vi "Lab Panel V4.83.vi"() -> ()   [LabVIEW 2013] (continued)
                            n1243 = local write "data file error"(w2114) -> ()
                          }
                          frame #1 {
                            n1244 = Bundle(cluster=w2115, "STATUS"="T-RISE PASS") -> (w2117:T4)  [unwired: 2 in]
                            n1245 = local write "RESULT LAB03-1"(TRUE) -> ()
                            n1246 = local write "DISP LAB03-1"(w2117) -> ()
                          }
                        }
                      }
                      frame False {
                      }
                    }
                  }
                }
              }
              frame #5 {
                # "LAB03-2"
                n1247 = Equal?(x=w2120, y=2) -> (x = y?=w2123:bool)
                n1248 = local read "DISP LAB03-2"() -> (w2125:T4)
                n1249 = Unbundle(w2125) -> ("STATUS"=w2126:string)  [unwired: 2 out]
                n1250 = Equal?(x=w2126, y="RUN") -> (x = y?=w2122:bool)
                n1251 = And(x=w2122, y=w2123) -> (x .and. y?=w2121:bool)
                n1252 = case shown="True" w2121 {
                  tunnel: w2125 -> [_ w2129]
                  tunnel: w2119 -> [_ w2132]
                  frame False {
                  }
                  frame True {
                    n1253 = local read "SET LAB03-2"() -> (w2131:T5)
                    n1254 = local read "TDMS LAB03-2"() -> (w2128:refnum<k34>)
                    n1255 = Unbundle(w2129) -> ("CYCLE"=w2133:dbl)  [unwired: 2 out]
                    n1256 = Unbundle(w2131) -> ("T-RISE mins"=w2130:dbl)  [unwired: 4 out]
                    n1257 = Greater Or Equal?(x=w2133, y=w2132) -> (x >= y?=w2134:bool)
                    n1258 = case shown="True" w2134 {
                      tunnel: w2130 -> [w2137 _]
                      tunnel: w2129 -> [w2136 _]
                      tunnel: w2128 -> [w2135 _]
                      frame True {
                        n1259 = stacked-sequence {
                          tunnel: w2137 -> [w2140 _]
                          tunnel: w2136 -> [_ w2145]
                          tunnel: w2135 -> [w2138 _]
                          frame #0 {
                            n1260 = Build Array("T-RISE") -> (w2142:string[])
                            n1261 = Build Array(w2140) -> (w2141:dbl[])
                            n1262 = TDMS Write(0:w2138, 5:"TEST PASS", 7:w2142, 9:w2141) -> (15:w2144:errorcluster)  [unwired: 2 in, 3 out]
                            n1263 = local write "data file error"(w2144) -> ()
                          }
                          frame #1 {
                            n1264 = Bundle(cluster=w2145, "STATUS"="T-RISE PASS") -> (w2147:T4)  [unwired: 2 in]
                            n1265 = local write "RESULT LAB03-2"(TRUE) -> ()
                            n1266 = local write "DISP LAB03-2"(w2147) -> ()
                          }
                        }
                      }
                      frame False {
                      }
                    }
                  }
                }
              }
              frame #6 {
                # "LAB04-1"
                n1267 = Equal?(x=w2150, y=2) -> (x = y?=w2153:bool)
                n1268 = local read "DISP LAB04-1"() -> (w2155:T4)
                n1269 = Unbundle(w2155) -> ("STATUS"=w2156:string)  [unwired: 2 out]
                n1270 = Equal?(x=w2156, y="RUN") -> (x = y?=w2152:bool)
                n1271 = And(x=w2152, y=w2153) -> (x .and. y?=w2151:bool)
                n1272 = case shown="True" w2151 {
                  tunnel: w2155 -> [_ w2159]
                  tunnel: w2149 -> [_ w2162]
                  frame False {
                  }
                  frame True {
                    n1273 = local read "SET LAB04-1"() -> (w2161:T5)
                    n1274 = local read "TDMS LAB04-1"() -> (w2158:refnum<k34>)
                    n1275 = Unbundle(w2159) -> ("CYCLE"=w2163:dbl)  [unwired: 2 out]
                    n1276 = Unbundle(w2161) -> ("T-RISE mins"=w2160:dbl)  [unwired: 4 out]
                    n1277 = Greater Or Equal?(x=w2163, y=w2162) -> (x >= y?=w2164:bool)
                    n1278 = case shown="True" w2164 {
                      tunnel: w2160 -> [w2167 _]
                      tunnel: w2159 -> [w2166 _]
                      tunnel: w2158 -> [w2165 _]
                      frame True {
                        n1279 = stacked-sequence {
                          tunnel: w2167 -> [w2170 _]
                          tunnel: w2166 -> [_ w2175]
                          tunnel: w2165 -> [w2168 _]
                          frame #0 {
                            n1280 = Build Array("T-RISE") -> (w2172:string[])
                            n1281 = Build Array(w2170) -> (w2171:dbl[])
                            n1282 = TDMS Write(0:w2168, 5:"TEST PASS", 7:w2172, 9:w2171) -> (15:w2174:errorcluster)  [unwired: 2 in, 3 out]
                            n1283 = local write "data file error"(w2174) -> ()
                          }
                          frame #1 {
                            n1284 = Bundle(cluster=w2175, "STATUS"="T-RISE PASS") -> (w2177:T4)  [unwired: 2 in]
                            n1285 = local write "RESULT LAB04-1"(TRUE) -> ()
                            n1286 = local write "DISP LAB04-1"(w2177) -> ()
                          }
                        }
                      }
                      frame False {
                      }
                    }
                  }
                }
              }
              frame #7 {
                # "LAB04-2"
                n1287 = Equal?(x=w2180, y=2) -> (x = y?=w2183:bool)
                n1288 = local read "DISP LAB04-2"() -> (w2185:T4)
                n1289 = Unbundle(w2185) -> ("STATUS"=w2186:string)  [unwired: 2 out]
                n1290 = Equal?(x=w2186, y="RUN") -> (x = y?=w2182:bool)
                n1291 = And(x=w2182, y=w2183) -> (x .and. y?=w2181:bool)
                n1292 = case shown="True" w2181 {
                  tunnel: w2185 -> [_ w2189]
                  tunnel: w2179 -> [_ w2192]
                  frame False {
                  }
                  frame True {
                    n1293 = local read "SET LAB04-2"() -> (w2191:T5)
                    n1294 = local read "TDMS LAB04-2"() -> (w2188:refnum<k34>)
                    n1295 = Unbundle(w2189) -> ("CYCLE"=w2193:dbl)  [unwired: 2 out]
                    n1296 = Unbundle(w2191) -> ("T-RISE mins"=w2190:dbl)  [unwired: 4 out]
                    n1297 = Greater Or Equal?(x=w2193, y=w2192) -> (x >= y?=w2194:bool)
                    n1298 = case shown="True" w2194 {
                      tunnel: w2190 -> [w2197 _]
                      tunnel: w2189 -> [w2196 _]
                      tunnel: w2188 -> [w2195 _]
                      frame True {
                        n1299 = stacked-sequence {
                          tunnel: w2197 -> [w2200 _]
                          tunnel: w2196 -> [_ w2205]
                          tunnel: w2195 -> [w2198 _]
                          frame #0 {
                            n1300 = Build Array("T-RISE") -> (w2202:string[])
                            n1301 = Build Array(w2200) -> (w2201:dbl[])
                            n1302 = TDMS Write(0:w2198, 5:"TEST PASS", 7:w2202, 9:w2201) -> (15:w2204:errorcluster)  [unwired: 2 in, 3 out]
                            n1303 = local write "data file error"(w2204) -> ()
                          }
                          frame #1 {
                            n1304 = Bundle(cluster=w2205, "STATUS"="T-RISE PASS") -> (w2207:T4)  [unwired: 2 in]
                            n1305 = local write "RESULT LAB04-2"(TRUE) -> ()
                            n1306 = local write "DISP LAB04-2"(w2207) -> ()
                          }
                        }
                      }
                      frame False {
                      }
                    }
                  }
                }
              }
              frame #8 {
                # "LAB05-1"
                n1307 = Equal?(x=w2210, y=2) -> (x = y?=w2213:bool)
                n1308 = local read "DISP LAB05-1"() -> (w2215:T4)
                n1309 = Unbundle(w2215) -> ("STATUS"=w2216:string)  [unwired: 2 out]
                n1310 = Equal?(x=w2216, y="RUN") -> (x = y?=w2212:bool)
                n1311 = And(x=w2212, y=w2213) -> (x .and. y?=w2211:bool)
                n1312 = case shown="True" w2211 {
                  tunnel: w2215 -> [_ w2219]
                  tunnel: w2209 -> [_ w2222]
                  frame False {
                  }
                  frame True {
                    n1313 = local read "SET LAB05-1"() -> (w2221:T5)
                    n1314 = local read "TDMS LAB05-1"() -> (w2218:refnum<k34>)
                    n1315 = Unbundle(w2219) -> ("CYCLE"=w2223:dbl)  [unwired: 2 out]
                    n1316 = Unbundle(w2221) -> ("T-RISE mins"=w2220:dbl)  [unwired: 4 out]
                    n1317 = Greater Or Equal?(x=w2223, y=w2222) -> (x >= y?=w2224:bool)
                    n1318 = case shown="True" w2224 {
                      tunnel: w2220 -> [w2227 _]
                      tunnel: w2219 -> [w2226 _]
                      tunnel: w2218 -> [w2225 _]
                      frame True {
                        n1319 = stacked-sequence {
                          tunnel: w2227 -> [w2230 _]
                          tunnel: w2226 -> [_ w2235]
                          tunnel: w2225 -> [w2228 _]
                          frame #0 {
                            n1320 = Build Array("T-RISE") -> (w2232:string[])
                            n1321 = Build Array(w2230) -> (w2231:dbl[])
                            n1322 = TDMS Write(0:w2228, 5:"TEST PASS", 7:w2232, 9:w2231) -> (15:w2234:errorcluster)  [unwired: 2 in, 3 out]
                            n1323 = local write "data file error"(w2234) -> ()
                          }
                          frame #1 {
                            n1324 = Bundle(cluster=w2235, "STATUS"="T-RISE PASS") -> (w2237:T4)  [unwired: 2 in]
                            n1325 = local write "RESULT LAB05-1"(TRUE) -> ()
                            n1326 = local write "DISP LAB05-1"(w2237) -> ()
                          }
                        }
                      }
                      frame False {
                      }
                    }
                  }
                }
              }
              frame #9 {
                # "LAB05-2"
                n1327 = Equal?(x=w2240, y=2) -> (x = y?=w2243:bool)
                n1328 = local read "DISP LAB05-2"() -> (w2245:T4)
                n1329 = Unbundle(w2245) -> ("STATUS"=w2246:string)  [unwired: 2 out]
                n1330 = Equal?(x=w2246, y="RUN") -> (x = y?=w2242:bool)
                n1331 = And(x=w2242, y=w2243) -> (x .and. y?=w2241:bool)
                n1332 = case shown="True" w2241 {
                  tunnel: w2245 -> [_ w2249]
                  tunnel: w2239 -> [_ w2252]
                  frame False {
                  }
                  frame True {
                    n1333 = local read "SET LAB05-2"() -> (w2251:T5)
                    n1334 = local read "TDMS LAB05-2"() -> (w2248:refnum<k34>)
                    n1335 = Unbundle(w2249) -> ("CYCLE"=w2253:dbl)  [unwired: 2 out]
                    n1336 = Unbundle(w2251) -> ("T-RISE mins"=w2250:dbl)  [unwired: 4 out]
                    n1337 = Greater Or Equal?(x=w2253, y=w2252) -> (x >= y?=w2254:bool)
                    n1338 = case shown="True" w2254 {
                      tunnel: w2250 -> [w2257 _]
                      tunnel: w2249 -> [w2256 _]
                      tunnel: w2248 -> [w2255 _]
                      frame True {
                        n1339 = stacked-sequence {
                          tunnel: w2257 -> [w2260 _]
                          tunnel: w2256 -> [_ w2265]
                          tunnel: w2255 -> [w2258 _]
                          frame #0 {
                            n1340 = Build Array("T-RISE") -> (w2262:string[])
                            n1341 = Build Array(w2260) -> (w2261:dbl[])
                            n1342 = TDMS Write(0:w2258, 5:"TEST PASS", 7:w2262, 9:w2261) -> (15:w2264:errorcluster)  [unwired: 2 in, 3 out]
                            n1343 = local write "data file error"(w2264) -> ()
                          }
                          frame #1 {
                            n1344 = Bundle(cluster=w2265, "STATUS"="T-RISE PASS") -> (w2267:T4)  [unwired: 2 in]
                            n1345 = local write "RESULT LAB05-2"(TRUE) -> ()
                            n1346 = local write "DISP LAB05-2"(w2267) -> ()
                          }
                        }
                      }
                      frame False {
                      }
                    }
                  }
                }
              }
            }
          }
          frame #6 {
            # "end test & close test files"
            n1347 = stacked-sequence {
              tunnel: w2278 -> [_ _ _ _ _ _ _ _ _ _]
              tunnel: w2279 -> [_ _ _ _ _ _ _ _ _ _]
              tunnel: w2277 -> [_ _ _ _ _ _ _ _ _ _]
              tunnel: w2276 -> [_ _ _ _ _ _ _ _ _ _]
              tunnel: w2275 -> [_ _ _ _ _ _ _ _ _ _]
              tunnel: w2274 -> [_ _ _ _ _ _ _ _ _ _]
              tunnel: w2273 -> [_ _ _ _ _ _ _ _ _ _]
              tunnel: w2272 -> [_ _ _ _ _ _ _ _ _ _]
              tunnel: w2271 -> [_ _ _ _ _ _ _ _ _ _]
              tunnel: w2270 -> [_ _ _ _ _ _ _ _ _ _]
              frame #0 {
                # "LAB01-1"
                n1348 = local read "DISP LAB01-1"() -> (w2283:T4)
                n1349 = local read "run lab01-1"() -> (w2280:bool)
                n1350 = local read "TDMS LAB01-1"() -> (w2281:refnum<k34>)
                n1351 = Unbundle(w2283) -> ("CYCLE"=w2284:dbl, "STATUS"=w2282:string)  [unwired: 1 out]
                n1352 = case shown="True" w2280 {
                  tunnel: w2284 -> [_ w2285]
                  tunnel: w2283 -> [_ w2288]
                  tunnel: w2282 -> [_ w2287]
                  tunnel: w2281 -> [_ w2286]
                  frame False {
                  }
                  frame True {
                    n1353 = Not Equal?(x=w2287, y="RUN") -> (x != y?=w2289:bool)
                    n1354 = Greater?(x=w2285, y=2.0) -> (0:w2291:bool)
                    n1355 = And(x=w2291, y=w2289) -> (x .and. y?=w2290:bool)
                    n1356 = case shown="True" w2290 {
                      tunnel: w2288 -> [_ w2296]
                      tunnel: w2286 -> [_ w2295]
                      tunnel: w2285 -> [_ w2294]
                      frame False {
                      }
                      frame True {
                        n1357 = stacked-sequence {
                          tunnel: w2296 -> [w2300 _ _]
                          tunnel: w2295 -> [_ w2302 _]
                          tunnel: w2294 -> [_ _ _]
                          frame #0 {
                            w2297 = FALSE
                            n1358 = local write "mail control"("END") -> ()
                            n1359 = Bundle(cluster=w2300) -> (w2299:T4)  [unwired: 3 in]
                            n1360 = local write "DISP LAB01-1"(w2299) -> ()
                            n1361 = local write "O/I  LAB01-1"(w2297) -> ()
                            n1362 = local write "run lab01-1"(w2297) -> ()
                            n1363 = local write "RUN LAB01-1"(w2297) -> ()
                          }
                          frame #1 {
                            n1364 = TDMS Close(11:w2302) -> (0:w2301:errorcluster)  [unwired: 1 in, 1 out]
                            n1365 = local write "data file error"(w2301) -> ()
                          }
                          frame #2 {
                            n1366 = stacked-sequence {
                              tunnel: "LAB01-1" -> [w2305 w2307]
                              frame #0 {
                                n1367 = call "sub vi - defrag tdms v1.vi"("panel id"=w2305) -> ("error out"=w2304:errorcluster)  [unwired: 10 in]
                                n1368 = local write "data file error"(w2304) -> ()
                              }
                              frame #1 {
                                n1369 = call "Save data file to network drive v2.vi"("panel id"=w2307) -> ("network file save error"=w2306:errorcluster)  [unwired: 9 in, 1 out]
                                n1370 = local write "data file error"(w2306) -> ()
                              }
                            }
                          }
                        }
                      }
                    }
                  }
                }
              }
              frame #1 {
                # "LAB01-2"
                n1371 = local read "run lab01-2"() -> (w2308:bool)
                n1372 = case shown="True" w2308 {
                  frame False {
                  }
                  frame True {
                    n1373 = local read "DISP LAB01-2"() -> (w2315:T4)
                    n1374 = local read "TDMS LAB01-2"() -> (w2314:refnum<k34>)
                    n1375 = Unbundle(w2315) -> ("CYCLE"=w2309:dbl, "STATUS"=w2316:string)  [unwired: 1 out]
                    n1376 = Not Equal?(x=w2316, y="RUN") -> (x != y?=w2311:bool)
                    n1377 = Greater?(x=w2309, y=2.0) -> (0:w2312:bool)
                    n1378 = And(x=w2312, y=w2311) -> (x .and. y?=w2310:bool)
                    n1379 = case shown="True" w2310 {
                      tunnel: w2315 -> [_ w2320]
                      tunnel: w2314 -> [_ w2319]
                      tunnel: w2309 -> [_ w2318]
                      frame False {
                      }
                      frame True {
                        n1380 = stacked-sequence {
                          tunnel: w2320 -> [w2323 _ _]
                          tunnel: w2319 -> [_ w2325 _]
                          tunnel: w2318 -> [_ _ _]
                          frame #0 {
                            w2321 = FALSE
                            n1381 = local write "mail control"("END") -> ()
                            n1382 = Bundle(cluster=w2323) -> (w2324:T4)  [unwired: 3 in]
                            n1383 = local write "RUN LAB01-2"(w2321) -> ()
                            n1384 = local write "run lab01-2"(w2321) -> ()
                            n1385 = local write "O/I  LAB01-2"(w2321) -> ()
                            n1386 = local write "DISP LAB01-2"(w2324) -> ()
                          }
                          frame #1 {
                            n1387 = TDMS Close(11:w2325) -> (0:w2326:errorcluster)  [unwired: 1 in, 1 out]
                            n1388 = local write "data file error"(w2326) -> ()
                          }
                          frame #2 {
                            n1389 = stacked-sequence {
                              tunnel: "LAB01-2" -> [w2329 w2331]
                              frame #0 {
                                n1390 = call "sub vi - defrag tdms v1.vi"("panel id"=w2329) -> ("error out"=w2328:errorcluster)  [unwired: 10 in]
                                n1391 = local write "data file error"(w2328) -> ()
                              }
                              frame #1 {
                                n1392 = call "Save data file to network drive v2.vi"("panel id"=w2331) -> ("network file save error"=w2330:errorcluster)  [unwired: 9 in, 1 out]
                                n1393 = local write "data file error"(w2330) -> ()
                              }
                            }
                          }
                        }
                      }
                    }
                  }
                }
              }
              frame #2 {
                # "LAB02-1"
                n1394 = local read "run lab02-1"() -> (w2332:bool)
                n1395 = case shown="True" w2332 {
                  frame False {
                  }
                  frame True {
                    n1396 = local read "DISP LAB02-1"() -> (w2339:T4)
                    n1397 = Unbundle(w2339) -> ("CYCLE"=w2335:dbl, "STATUS"=w2340:string)  [unwired: 1 out]
                    n1398 = local read "TDMS LAB02-1"() -> (w2338:refnum<k34>)
                    n1399 = Not Equal?(x=w2340, y="RUN") -> (x != y?=w2334:bool)
                    n1400 = Greater?(x=w2335, y=2.0) -> (0:w2336:bool)
                    n1401 = And(x=w2336, y=w2334) -> (x .and. y?=w2333:bool)
                    n1402 = case shown="True" w2333 {
                      tunnel: w2339 -> [_ w2343]
                      tunnel: w2338 -> [_ w2342]
                      frame False {
                      }
                      frame True {
                        n1403 = stacked-sequence {
                          tunnel: w2343 -> [w2346 _ _]
                          tunnel: w2342 -> [_ w2348 _]
                          frame #0 {
                            w2344 = FALSE
                            n1404 = local write "mail control"("END") -> ()
                            n1405 = Bundle(cluster=w2346) -> (w2347:T4)  [unwired: 3 in]
                            n1406 = local write "O/I  LAB02-1"(w2344) -> ()
                            n1407 = local write "RUN LAB02-1"(w2344) -> ()
                            n1408 = local write "run lab02-1"(w2344) -> ()
                            n1409 = local write "DISP LAB02-1"(w2347) -> ()
                          }
                          frame #1 {
                            n1410 = TDMS Close(11:w2348) -> (0:w2349:errorcluster)  [unwired: 1 in, 1 out]
                            n1411 = local write "data file error"(w2349) -> ()
                          }
                          frame #2 {
                            n1412 = stacked-sequence {
                              tunnel: "LAB02-1" -> [w2352 w2354]
                              frame #0 {
                                n1413 = call "sub vi - defrag tdms v1.vi"("panel id"=w2352) -> ("error out"=w2351:errorcluster)  [unwired: 10 in]
                                n1414 = local write "data file error"(w2351) -> ()
                              }
                              frame #1 {
                                n1415 = call "Save data file to network drive v2.vi"("panel id"=w2354) -> ("network file save error"=w2353:errorcluster)  [unwired: 9 in, 1 out]
                                n1416 = local write "data file error"(w2353) -> ()
                              }
                            }
                          }
                        }
                      }
                    }
                  }
                }
              }
              frame #3 {
                # "LAB02-2"
                n1417 = local read "run lab02-2"() -> (w2355:bool)
                n1418 = case shown="True" w2355 {
                  frame False {
                  }
                  frame True {
                    n1419 = local read "DISP LAB02-2"() -> (w2362:T4)
                    n1420 = local read "TDMS LAB02-2"() -> (w2361:refnum<k34>)
                    n1421 = Unbundle(w2362) -> ("CYCLE"=w2358:dbl, "STATUS"=w2363:string)  [unwired: 1 out]
                    n1422 = Not Equal?(x=w2363, y="RUN") -> (x != y?=w2357:bool)
                    n1423 = Greater?(x=w2358, y=2.0) -> (0:w2359:bool)
                    n1424 = And(x=w2359, y=w2357) -> (x .and. y?=w2356:bool)
                    n1425 = case shown="True" w2356 {
                      tunnel: w2362 -> [_ w2366]
                      tunnel: w2361 -> [_ w2365]
                      frame False {
                      }
                      frame True {
                        n1426 = stacked-sequence {
                          tunnel: w2366 -> [w2369 _ _]
                          tunnel: w2365 -> [_ w2371 _]
                          frame #0 {
                            w2367 = FALSE
                            n1427 = local write "mail control"("END") -> ()
                            n1428 = Bundle(cluster=w2369) -> (w2370:T4)  [unwired: 3 in]
                            n1429 = local write "O/I  LAB02-2"(w2367) -> ()
                            n1430 = local write "run lab02-2"(w2367) -> ()
                            n1431 = local write "RUN LAB02-2"(w2367) -> ()
                            n1432 = local write "DISP LAB02-2"(w2370) -> ()
                          }
                          frame #1 {
                            n1433 = TDMS Close(11:w2371) -> (0:w2372:errorcluster)  [unwired: 1 in, 1 out]
                            n1434 = local write "data file error"(w2372) -> ()
                          }
                          frame #2 {
                            n1435 = stacked-sequence {
                              tunnel: "LAB02-2" -> [w2375 w2377]
                              frame #0 {
                                n1436 = call "sub vi - defrag tdms v1.vi"("panel id"=w2375) -> ("error out"=w2374:errorcluster)  [unwired: 10 in]
                                n1437 = local write "data file error"(w2374) -> ()
                              }
                              frame #1 {
                                n1438 = call "Save data file to network drive v2.vi"("panel id"=w2377) -> ("network file save error"=w2376:errorcluster)  [unwired: 9 in, 1 out]
                                n1439 = local write "data file error"(w2376) -> ()
                              }
                            }
                          }
                        }
                      }
                    }
                  }
                }
              }
              frame #4 {
                # "LAB03-1"
                n1440 = local read "run lab03-1"() -> (w2378:bool)
                n1441 = case shown="True" w2378 {
                  frame False {
                  }
                  frame True {
                    n1442 = local read "DISP LAB03-1"() -> (w2385:T4)
                    n1443 = local read "TDMS LAB03-1"() -> (w2384:refnum<k34>)
                    n1444 = Unbundle(w2385) -> ("CYCLE"=w2381:dbl, "STATUS"=w2386:string)  [unwired: 1 out]
                    n1445 = Not Equal?(x=w2386, y="RUN") -> (x != y?=w2380:bool)
                    n1446 = Greater?(x=w2381, y=2.0) -> (0:w2382:bool)
                    n1447 = And(x=w2382, y=w2380) -> (x .and. y?=w2379:bool)
                    n1448 = case shown="True" w2379 {
                      tunnel: w2385 -> [_ w2389]
                      tunnel: w2384 -> [_ w2388]
                      frame False {
                      }
                      frame True {
                        n1449 = stacked-sequence {
                          tunnel: w2389 -> [w2392 _ _]
                          tunnel: w2388 -> [_ w2394 _]
                          frame #0 {
                            w2390 = FALSE
                            n1450 = local write "mail control"("END") -> ()
                            n1451 = Bundle(cluster=w2392) -> (w2393:T4)  [unwired: 3 in]
                            n1452 = local write "O/I  LAB03-1"(w2390) -> ()
                            n1453 = local write "run lab03-1"(w2390) -> ()
                            n1454 = local write "RUN LAB03-1"(w2390) -> ()
                            n1455 = local write "DISP LAB03-1"(w2393) -> ()
                          }
                          frame #1 {
                            n1456 = TDMS Close(11:w2394) -> (0:w2395:errorcluster)  [unwired: 1 in, 1 out]
                            n1457 = local write "data file error"(w2395) -> ()
                          }
                          frame #2 {
                            n1458 = stacked-sequence {
                              tunnel: "LAB03-1" -> [w2398 w2400]
                              frame #0 {
                                n1459 = call "sub vi - defrag tdms v1.vi"("panel id"=w2398) -> ("error out"=w2397:errorcluster)  [unwired: 10 in]
                                n1460 = local write "data file error"(w2397) -> ()
                              }
                              frame #1 {
                                n1461 = call "Save data file to network drive v2.vi"("panel id"=w2400) -> ("network file save error"=w2399:errorcluster)  [unwired: 9 in, 1 out]
                                n1462 = local write "data file error"(w2399) -> ()
                              }
                            }
                          }
                        }
                      }
                    }
                  }
                }
              }
              frame #5 {
                # "LAB03-2"
                n1463 = local read "run lab03-2"() -> (w2401:bool)
                n1464 = case shown="True" w2401 {
                  frame False {
                  }
                  frame True {
                    n1465 = local read "DISP LAB03-2"() -> (w2408:T4)
                    n1466 = Unbundle(w2408) -> ("CYCLE"=w2404:dbl, "STATUS"=w2409:string)  [unwired: 1 out]
                    n1467 = local read "TDMS LAB03-2"() -> (w2407:refnum<k34>)
                    n1468 = Not Equal?(x=w2409, y="RUN") -> (x != y?=w2403:bool)
                    n1469 = Greater?(x=w2404, y=2.0) -> (0:w2405:bool)
                    n1470 = And(x=w2405, y=w2403) -> (x .and. y?=w2402:bool)
                    n1471 = case shown="True" w2402 {
                      tunnel: w2408 -> [_ w2412]
                      tunnel: w2407 -> [_ w2411]
                      frame False {
                      }
                      frame True {
                        n1472 = stacked-sequence {
                          tunnel: w2412 -> [w2415 _ _]
                          tunnel: w2411 -> [_ w2417 _]
                          frame #0 {
                            w2413 = FALSE
                            n1473 = local write "mail control"("END") -> ()
                            n1474 = Bundle(cluster=w2415) -> (w2416:T4)  [unwired: 3 in]
                            n1475 = local write "RUN LAB03-2"(w2413) -> ()
                            n1476 = local write "O/I  LAB03-2"(w2413) -> ()
                            n1477 = local write "DISP LAB03-2"(w2416) -> ()
                            n1478 = local write "run lab03-2"(w2413) -> ()
                          }
                          frame #1 {
                            n1479 = TDMS Close(11:w2417) -> (0:w2418:errorcluster)  [unwired: 1 in, 1 out]
                            n1480 = local write "data file error"(w2418) -> ()
                          }
                          frame #2 {
                            n1481 = stacked-sequence {
                              tunnel: "LAB03-2" -> [w2421 w2423]
                              frame #0 {
                                n1482 = call "sub vi - defrag tdms v1.vi"("panel id"=w2421) -> ("error out"=w2420:errorcluster)  [unwired: 10 in]
                                n1483 = local write "data file error"(w2420) -> ()
                              }
                              frame #1 {
                                n1484 = call "Save data file to network drive v2.vi"("panel id"=w2423) -> ("network file save error"=w2422:errorcluster)  [unwired: 9 in, 1 out]
                                n1485 = local write "data file error"(w2422) -> ()
                              }
                            }
                          }
                        }
                      }
                    }
                  }
                }
              }
              frame #6 {
                # "LAB04-1"
                n1486 = local read "run lab04-1"() -> (w2424:bool)
                n1487 = case shown="True" w2424 {
                  frame False {
                  }
                  frame True {
                    n1488 = local read "DISP LAB04-1"() -> (w2431:T4)
                    n1489 = Unbundle(w2431) -> ("CYCLE"=w2427:dbl, "STATUS"=w2432:string)  [unwired: 1 out]
                    n1490 = local read "TDMS LAB04-1"() -> (w2430:refnum<k34>)
                    n1491 = Not Equal?(x=w2432, y="RUN") -> (x != y?=w2426:bool)
                    n1492 = Greater?(x=w2427, y=2.0) -> (0:w2428:bool)
                    n1493 = And(x=w2428, y=w2426) -> (x .and. y?=w2425:bool)
                    n1494 = case shown="True" w2425 {
                      tunnel: w2431 -> [_ w2435]
                      tunnel: w2430 -> [_ w2434]
                      frame False {
                      }
                      frame True {
                        n1495 = stacked-sequence {
                          tunnel: w2435 -> [w2438 _ _]
                          tunnel: w2434 -> [_ w2440 _]
                          frame #0 {
                            w2436 = FALSE
                            n1496 = local write "mail control"("END") -> ()
                            n1497 = Bundle(cluster=w2438) -> (w2439:T4)  [unwired: 3 in]
                            n1498 = local write "RUN LAB04-1"(w2436) -> ()
                            n1499 = local write "O/I  LAB04-1"(w2436) -> ()
                            n1500 = local write "run lab04-1"(w2436) -> ()
                            n1501 = local write "DISP LAB04-1"(w2439) -> ()
                          }
                          frame #1 {
                            n1502 = TDMS Close(11:w2440) -> (0:w2441:errorcluster)  [unwired: 1 in, 1 out]
                            n1503 = local write "data file error"(w2441) -> ()
                          }
                          frame #2 {
                            n1504 = stacked-sequence {
                              tunnel: "LAB04-1" -> [w2444 w2446]
                              frame #0 {
                                n1505 = call "sub vi - defrag tdms v1.vi"("panel id"=w2444) -> ("error out"=w2443:errorcluster)  [unwired: 10 in]
                                n1506 = local write "data file error"(w2443) -> ()
                              }
                              frame #1 {
                                n1507 = call "Save data file to network drive v2.vi"("panel id"=w2446) -> ("network file save error"=w2445:errorcluster)  [unwired: 9 in, 1 out]
                                n1508 = local write "data file error"(w2445) -> ()
                              }
                            }
                          }
                        }
                      }
                    }
                  }
                }
              }
              frame #7 {
                # "LAB04-2"
                n1509 = local read "run lab04-2"() -> (w2447:bool)
                n1510 = case shown="True" w2447 {
                  frame False {
                  }
                  frame True {
                    n1511 = local read "DISP LAB04-2"() -> (w2454:T4)
                    n1512 = Unbundle(w2454) -> ("CYCLE"=w2450:dbl, "STATUS"=w2455:string)  [unwired: 1 out]
                    n1513 = Not Equal?(x=w2455, y="RUN") -> (x != y?=w2449:bool)
                    n1514 = local read "TDMS LAB04-2"() -> (w2453:refnum<k34>)
                    n1515 = Greater?(x=w2450, y=2.0) -> (0:w2451:bool)
                    n1516 = And(x=w2451, y=w2449) -> (x .and. y?=w2448:bool)
                    n1517 = case shown="True" w2448 {
                      tunnel: w2454 -> [_ w2458]
                      tunnel: w2453 -> [_ w2457]
                      frame False {
                      }
                      frame True {
                        n1518 = stacked-sequence {
                          tunnel: w2458 -> [w2461 _ _]
                          tunnel: w2457 -> [_ w2463 _]
                          frame #0 {
                            w2459 = FALSE
                            n1519 = local write "mail control"("END") -> ()
                            n1520 = Bundle(cluster=w2461) -> (w2462:T4)  [unwired: 3 in]
                            n1521 = local write "O/I  LAB04-2"(w2459) -> ()
                            n1522 = local write "RUN LAB04-2"(w2459) -> ()
                            n1523 = local write "run lab04-2"(w2459) -> ()
                            n1524 = local write "DISP LAB04-2"(w2462) -> ()
                          }
                          frame #1 {
                            n1525 = TDMS Close(11:w2463) -> (0:w2464:errorcluster)  [unwired: 1 in, 1 out]
                            n1526 = local write "data file error"(w2464) -> ()
                          }
                          frame #2 {
                            n1527 = stacked-sequence {
                              tunnel: "LAB04-2" -> [w2467 w2469]
                              frame #0 {
                                n1528 = call "sub vi - defrag tdms v1.vi"("panel id"=w2467) -> ("error out"=w2466:errorcluster)  [unwired: 10 in]
                                n1529 = local write "data file error"(w2466) -> ()
                              }
                              frame #1 {
                                n1530 = call "Save data file to network drive v2.vi"("panel id"=w2469) -> ("network file save error"=w2468:errorcluster)  [unwired: 9 in, 1 out]
                                n1531 = local write "data file error"(w2468) -> ()
                              }
                            }
                          }
                        }
                      }
                    }
                  }
                }
              }
              frame #8 {
                # "LAB05-1"
                n1532 = local read "run lab05-1"() -> (w2470:bool)
                n1533 = case shown="True" w2470 {
                  frame False {
                  }
                  frame True {
                    n1534 = local read "DISP LAB05-1"() -> (w2477:T4)
                    n1535 = Unbundle(w2477) -> ("CYCLE"=w2473:dbl, "STATUS"=w2478:string)  [unwired: 1 out]
                    n1536 = Not Equal?(x=w2478, y="RUN") -> (x != y?=w2472:bool)
                    n1537 = local read "TDMS LAB05-1"() -> (w2476:refnum<k34>)
                    n1538 = Greater?(x=w2473, y=2.0) -> (0:w2474:bool)
                    n1539 = And(x=w2474, y=w2472) -> (x .and. y?=w2471:bool)
                    n1540 = case shown="True" w2471 {
                      tunnel: w2477 -> [_ w2481]
                      tunnel: w2476 -> [_ w2480]
                      frame False {
                      }
                      frame True {
                        n1541 = stacked-sequence {
                          tunnel: w2481 -> [w2484 _ _]
                          tunnel: w2480 -> [_ w2486 _]
                          frame #0 {
                            w2482 = FALSE
                            n1542 = local write "mail control"("END") -> ()
                            n1543 = Bundle(cluster=w2484) -> (w2485:T4)  [unwired: 3 in]
                            n1544 = local write "O/I  LAB05-1"(w2482) -> ()
                            n1545 = local write "RUN LAB05-1"(w2482) -> ()
                            n1546 = local write "run lab05-1"(w2482) -> ()
                            n1547 = local write "DISP LAB05-1"(w2485) -> ()
                          }
                          frame #1 {
                            n1548 = TDMS Close(11:w2486) -> (0:w2487:errorcluster)  [unwired: 1 in, 1 out]
                            n1549 = local write "data file error"(w2487) -> ()
                          }
                          frame #2 {
                            n1550 = stacked-sequence {
                              tunnel: "LAB05-1" -> [w2490 w2492]
                              frame #0 {
                                n1551 = call "sub vi - defrag tdms v1.vi"("panel id"=w2490) -> ("error out"=w2489:errorcluster)  [unwired: 10 in]
                                n1552 = local write "data file error"(w2489) -> ()
                              }
                              frame #1 {
                                n1553 = call "Save data file to network drive v2.vi"("panel id"=w2492) -> ("network file save error"=w2491:errorcluster)  [unwired: 9 in, 1 out]
                                n1554 = local write "data file error"(w2491) -> ()
                              }
                            }
                          }
                        }
                      }
                    }
                  }
                }
              }
              frame #9 {
                # "LAB05-2"
                n1555 = local read "run lab05-2"() -> (w2493:bool)
                n1556 = case shown="True" w2493 {
                  frame False {
                  }
                  frame True {
                    n1557 = local read "DISP LAB05-2"() -> (w2500:T4)
                    n1558 = Unbundle(w2500) -> ("CYCLE"=w2496:dbl, "STATUS"=w2501:string)  [unwired: 1 out]
                    n1559 = Not Equal?(x=w2501, y="RUN") -> (x != y?=w2495:bool)
                    n1560 = local read "TDMS LAB05-2"() -> (w2499:refnum<k34>)
                    n1561 = Greater?(x=w2496, y=2.0) -> (0:w2497:bool)
                    n1562 = And(x=w2497, y=w2495) -> (x .and. y?=w2494:bool)
                    n1563 = case shown="True" w2494 {
                      tunnel: w2500 -> [_ w2504]
                      tunnel: w2499 -> [_ w2503]
                      frame False {
                      }
                      frame True {
                        n1564 = stacked-sequence {
                          tunnel: w2504 -> [w2507 _ _]
                          tunnel: w2503 -> [_ w2509 _]
                          frame #0 {
                            w2505 = FALSE
                            n1565 = local write "mail control"("END") -> ()
                            n1566 = Bundle(cluster=w2507) -> (w2508:T4)  [unwired: 3 in]
                            n1567 = local write "RUN LAB05-2"(w2505) -> ()
                            n1568 = local write "O/I  LAB05-2"(w2505) -> ()
                            n1569 = local write "run lab05-2"(w2505) -> ()
                            n1570 = local write "DISP LAB05-2"(w2508) -> ()
                          }
                          frame #1 {
                            n1571 = TDMS Close(11:w2509) -> (0:w2510:errorcluster)  [unwired: 1 in, 1 out]
                            n1572 = local write "data file error"(w2510) -> ()
                          }
                          frame #2 {
                            n1573 = stacked-sequence {
                              tunnel: "LAB05-2" -> [w2513 w2515]
                              frame #0 {
                                n1574 = call "sub vi - defrag tdms v1.vi"("panel id"=w2513) -> ("error out"=w2512:errorcluster)  [unwired: 10 in]
                                n1575 = local write "data file error"(w2512) -> ()
                              }
                              frame #1 {
                                n1576 = call "Save data file to network drive v2.vi"("panel id"=w2515) -> ("network file save error"=w2514:errorcluster)  [unwired: 9 in, 1 out]
                                n1577 = local write "data file error"(w2514) -> ()
                              }
                            }
                          }
                        }
                      }
                    }
                  }
                }
              }
            }
            n1578 = local read "Network Directory"() -> (w2269:path)
            n1579 = global write "Global 1.vi" "Network Drive"(w2269) -> ()
          }
          frame #7 {
            # "disable functions"
            n1580 = stacked-sequence {
              tunnel: w2525 -> [w2539 _ w2596]
              tunnel: w2524 -> [w2534 _ w2595]
              tunnel: w2523 -> [w2533 _ w2594]
              tunnel: w2522 -> [w2531 _ w2593]
              tunnel: w2521 -> [w2532 _ w2592]
              tunnel: w2520 -> [_ w2556 w2591]
              tunnel: w2519 -> [_ w2557 w2590]
              tunnel: w2518 -> [_ w2558 w2589]
              tunnel: w2517 -> [_ w2559 w2588]
              tunnel: w2516 -> [_ w2560 w2587]
              frame #0 {
                n1581 = Select(t=2, s=w2531, f=0) -> (s? t:f=w2527:i32)
                n1582 = Select(t=2, s=w2533, f=0) -> (s? t:f=w2528:i32)
                n1583 = Select(t=2, s=w2532, f=0) -> (s? t:f=w2526:i32)
                n1584 = Select(t=2, s=w2539, f=0) -> (s? t:f=w2530:i32)
                n1585 = Select(t=2, s=w2534, f=0) -> (s? t:f=w2529:i32)
                n1586 = property on="SELECT LAB02-2" class="RadioBtnsControl (strict)"("DisabledEnum"=w2527) -> ()  [unwired: 2 in, 2 out]
                n1587 = property on="SELECT LAB02-1" class="RadioBtnsControl (strict)"("DisabledEnum"=w2528) -> ()  [unwired: 2 in, 2 out]
                n1588 = property on="SELECT LAB03-1" class="RadioBtnsControl (strict)"("DisabledEnum"=w2526) -> ()  [unwired: 2 in, 2 out]
                n1589 = property on="SELECT LAB01-1" class="RadioBtnsControl (strict)"("DisabledEnum"=w2530) -> ()  [unwired: 2 in, 2 out]
                n1590 = property on="SELECT LAB01-2" class="RadioBtnsControl (strict)"("DisabledEnum"=w2529) -> ()  [unwired: 2 in, 2 out]
                n1591 = Not(x=w2539) -> (.not. x?=w2540:bool)
                n1592 = property on="RESULT LAB01-1" class="Bool (strict)"("Visible"=w2540) -> ()  [unwired: 2 in, 2 out]
                n1593 = Not(x=w2534) -> (.not. x?=w2538:bool)
                n1594 = Not(x=w2533) -> (.not. x?=w2537:bool)
                n1595 = Not(x=w2531) -> (.not. x?=w2536:bool)
                n1596 = property on="RESULT LAB01-2" class="Bool (strict)"("Visible"=w2538) -> ()  [unwired: 2 in, 2 out]
                n1597 = Not(x=w2532) -> (.not. x?=w2535:bool)
                n1598 = property on="RESULT LAB02-1" class="Bool (strict)"("Visible"=w2537) -> ()  [unwired: 2 in, 2 out]
                n1599 = property on="RESULT LAB02-2" class="Bool (strict)"("Visible"=w2536) -> ()  [unwired: 2 in, 2 out]
                n1600 = property on="RESULT LAB03-1" class="Bool (strict)"("Visible"=w2535) -> ()  [unwired: 2 in, 2 out]
                n1601 = property on="SET LAB01-1" class="Clust (strict)"("DisabledEnum"=w2530) -> ()  [unwired: 2 in, 2 out]
                n1602 = property on="SET LAB01-2" class="Clust (strict)"("DisabledEnum"=w2529) -> ()  [unwired: 2 in, 2 out]
                n1603 = property on="SET LAB02-1" class="Clust (strict)"("DisabledEnum"=w2528) -> ()  [unwired: 2 in, 2 out]
                n1604 = property on="SET LAB02-2" class="Clust (strict)"("DisabledEnum"=w2527) -> ()  [unwired: 2 in, 2 out]
                n1605 = property on="SET LAB03-1" class="Clust (strict)"("DisabledEnum"=w2526) -> ()  [unwired: 2 in, 2 out]
                n1606 = property on="O/I  LAB01-1" class="Bool (strict)"("DisabledEnum"=w2530) -> ()  [unwired: 2 in, 2 out]
                n1607 = property on="O/I  LAB01-2" class="Bool (strict)"("DisabledEnum"=w2529) -> ()  [unwired: 2 in, 2 out]
                n1608 = property on="O/I  LAB02-1" class="Bool (strict)"("DisabledEnum"=w2528) -> ()  [unwired: 2 in, 2 out]
                n1609 = property on="O/I  LAB02-2" class="Bool (strict)"("DisabledEnum"=w2527) -> ()  [unwired: 2 in, 2 out]
                n1610 = property on="O/I  LAB03-1" class="Bool (strict)"("DisabledEnum"=w2526) -> ()  [unwired: 2 in, 2 out]
              }
              frame #1 {
                n1611 = Select(t=2, s=w2560, f=0) -> (s? t:f=w2551:i32)
                n1612 = Select(t=2, s=w2559, f=0) -> (s? t:f=w2552:i32)
                n1613 = Select(t=2, s=w2556, f=0) -> (s? t:f=w2555:i32)
                n1614 = Select(t=2, s=w2557, f=0) -> (s? t:f=w2554:i32)
                n1615 = Select(t=2, s=w2558, f=0) -> (s? t:f=w2553:i32)
                n1616 = property on="SELECT LAB05-2" class="RadioBtnsControl (strict)"("DisabledEnum"=w2551) -> ()  [unwired: 2 in, 2 out]
                n1617 = property on="SELECT LAB05-1" class="RadioBtnsControl (strict)"("DisabledEnum"=w2552) -> ()  [unwired: 2 in, 2 out]
                n1618 = property on="SELECT LAB03-2" class="RadioBtnsControl (strict)"("DisabledEnum"=w2555) -> ()  [unwired: 2 in, 2 out]
                n1619 = property on="SELECT LAB04-1" class="RadioBtnsControl (strict)"("DisabledEnum"=w2554) -> ()  [unwired: 2 in, 2 out]
                n1620 = property on="SELECT LAB04-2" class="RadioBtnsControl (strict)"("DisabledEnum"=w2553) -> ()  [unwired: 2 in, 2 out]
                n1621 = property on="SET LAB05-2" class="Clust (strict)"("DisabledEnum"=w2551) -> ()  [unwired: 2 in, 2 out]
                n1622 = property on="SET LAB05-1" class="Clust (strict)"("DisabledEnum"=w2552) -> ()  [unwired: 2 in, 2 out]
